vi "ReferencedVariables_ReadReferencedVariable_6x8x6.vi"(0 "reference in":refnum<class>, 5 "error in (no error)":errorcluster) -> (14 "reference out":refnum<class>, 16 "ReplaceWithtypeDef":dbl, 19 "error out":errorcluster)   [LabVIEW 2010]
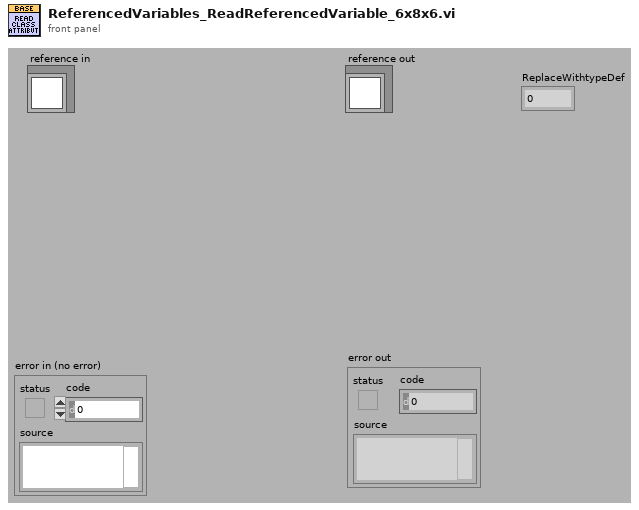
[diagram p1: front panel]
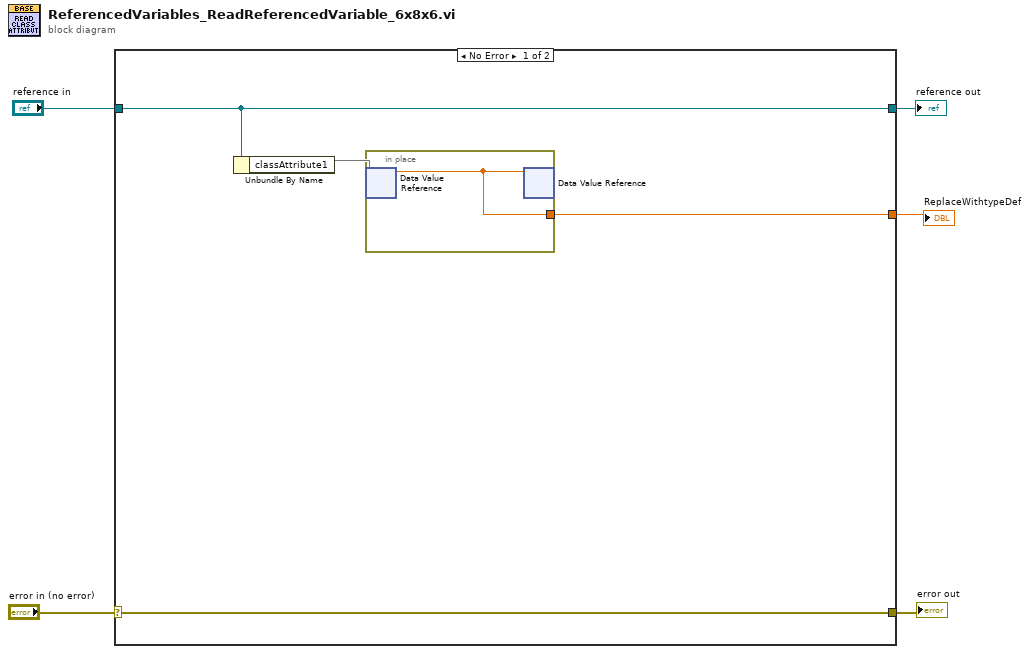
[diagram p0: block diagram]
diagram:
  n1 = case shown="No Error" "error in (no error)" {
    selector: "error in (no error)" -> [w7 w12]
    tunnel: [w7 w12] -> w4
    tunnel: [w8 w11] -> w2
    tunnel: "reference in" -> [w8 w11]
    tunnel: [w6 _] -> w1
    frame No Error {
      n2 = Unbundle By Name(w8) -> ("classAttribute1"=w9)
      n3 = in-place {
        in-place-border: [w10] -> w6
        n4 = in-place-dvr #1(w9) -> (w10:dbl)  [unwired: 1 out]
        n5 = in-place-dvr #1(w10) -> ()  [unwired: 2 out]
      }
    }
    frame Error {
    }
  }
  "error out" <- w4
  "reference out" <- w2
  "ReplaceWithtypeDef" <- w1
